vi "Rename Library And Class.vi"(4 "Post":string, 6 "Pre":string, 8 "error in":errorcluster, 9 "Rename Library File Path":path, 10 "Active Project":refnum<vi>) -> (0 "error out":errorcluster, 1 "Intermediate Library File Path":path)   [LabVIEW 2025, in "_Rename.lvlib" / "_Rename.lvclass"]
uses:
  _Rename.lvclass
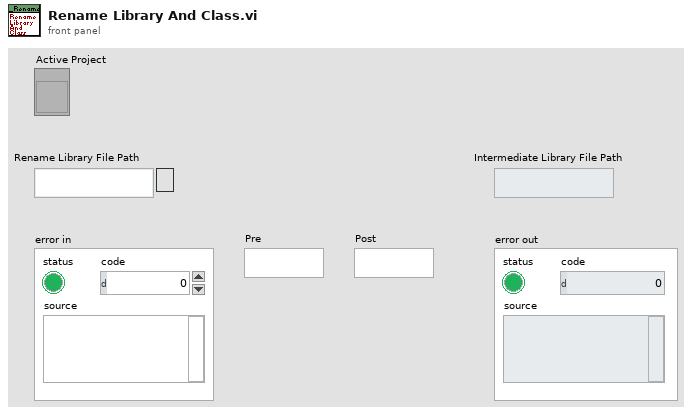
[diagram p1: front panel]
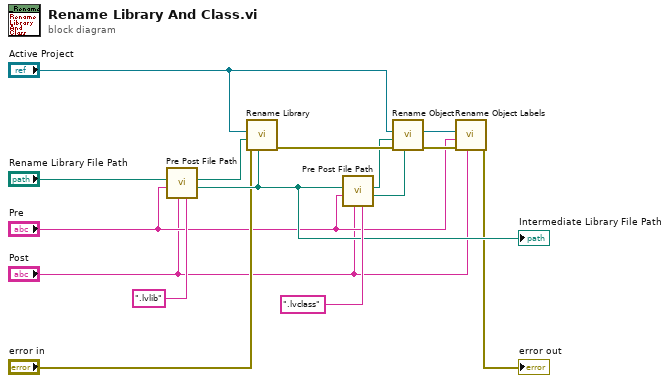
[diagram p0: block diagram]
diagram:
  n1 = call "Pre Post File Path.vi"("Extension"=".lvlib", "Post"="Post", "Pre"="Pre", "Rename Library File Path"="Rename Library File Path") -> ("Post File Path"=w7:path, "Pre File Path"=w11:path)  [unwired: 6 in]
  "Intermediate Library File Path" <- w7
  n2 = call "Rename Library.vi"("Rename Library File Path"=w7, "error in"="error in", "Name Library File Path"=w11, "Active Project"="Active Project") -> ("error out"=w12:errorcluster)  [unwired: 6 in, 1 out]
  n3 = call "Pre Post File Path.vi"("Extension"=".lvclass", "Post"="Post", "Pre"="Pre", "Rename Library File Path"=w7) -> ("Post File Path"=w8:path, "Pre File Path"=w9:path)  [unwired: 6 in]
  n4 = call "Rename Object.vi"("Post Object File Path"=w8, "error in"=w12, "Pre Object File Path"=w9, "Active Project"="Active Project") -> ("error out"=w15:errorcluster, "Object Ref"=w14:refnum<vi>)  [unwired: 6 in]
  n5 = call "Rename Object Labels.vi"("Post"="Post", "error in"=w15, "Pre"="Pre", "Class Ref"=w14) -> ("error out"=→"error out":errorcluster)  [unwired: 7 in]
